vi "event_trager_autoselect.vi"() -> ()   [LabVIEW 2013]
uses:
  <vilib>/silver_ctls/ArrayMatrixCluster/Real Matrix NI_Silver.ctl
  <vilib>/Utility/error.llb/DialogType.ctl
panel:
  in  "Warning Values":dbl[][](array[numeric])
  in  "Check":bool
  in  "repeat 2":dbl=4.0
  in  "interval/min 2":dbl=30.0
  in  "偏置电压":dbl=0.402 format="%0.2p"
  in  "明场周期":dbl=1.0 min=0.0 step=1.0
  in  "扫描起始电压":dbl=-1.0
  in  "振镜步长/um":dbl=0.6
  in  "Volume number":dbl=1.0 min=0.0 step=1.0
  in  "Image number":dbl=200.0
  in  "yx":dbl[][](array[numeric])=[[-0.228, -0.4392], [-0.7848, -0.8083], [-0.6027, 0.1673], [-0.8853, 0.367]]
  in  "waiting_stage/ms":i32=10
  in  "Scan Parameters":T1={"x start"=0.0, "y start"=0.0, "x end"=0.5, "y end"=0.5, "x number"=2.0, "y number"=2.0, "x step"=1.0, "y step"=1.0}
  in  "Stop":bool
  out "illum arr":bool[][](array[boolean])=[[TRUE, FALSE, FALSE, TRUE, FALSE], [FALSE, FALSE, FALSE, FALSE, TRUE], [FALSE, FALSE, FALSE, FALSE, FALSE], [FALSE, FALSE, FALSE, FALSE, TRUE], [FALSE, FALSE, FALSE, TRUE, FALSE]]
  out "total":dbl=4.0
  in  "index":dbl
  in  "exposure/ms":dbl=200.0
  in  "interval/min":dbl=1.0
  in  "repeat":dbl=1.0
  out "y num":dbl=0.772
  out "y target":dbl=-0.228
  out "x num":dbl=0.5608
  out "x target":dbl=-0.4392
  in  "auto compensation":bool
  out "z compensation":T2=[[-1.0, 3.300940438871473, 3.6018808777429463, 1.9028213166144192, 3.2037617554858926, 3.5047021943573657, 4.805642633228839, 7.106583072100312, 6.407523510971785, 5.708463949843258, 6.0094043887147315, 8.310344827586203, 7.611285266457677, 7.912225705329149, 8.213166144200624, 6.514106583072096, 9.81504702194357, 7.115987460815042, 8.416927899686517, 8.717868338557988, 9.018808777429463, 8.319749216300934, 8.620689655172407, 6.9216300940438815, 8.222570532915354, 9.523510971786827, 9.224451410658299, 9.125391849529773, 9.426332288401248, 9.72727272727272], [-0.701298701298701, -0.4017017465293328, -0.10210479175996456, 0.19749216300940375, 0.49708911777877196, 0.7966860725481403, 1.0962830273175084, 1.395879982086877, 1.6954769368562448, 1.9950738916256134, 2.2946708463949816, 2.59426780116435, 2.893864755933718, 3.193461710703086, 3.4930586654724545, 3.7926556202418227, 4.092252575011191, 4.3918495297805595, 4.691446484549928, 4.991043439319295, 5.290640394088664, 5.5902373488580315, 5.8898343036274, 6.189431258396769, 6.4890282131661365, 6.788625167935504, 7.088222122704873, 7.387819077474242, 7.68741603224361, 7.987012987012978], [1.7974025974025984, 2.8956560680698615, 5.193909538737125, 5.492163009404388, 7.790416480071652, 8.088669950738915, 10.38692342140618, 6.685176892073443, 8.983430362740705, 8.28168383340797, 8.579937304075234, 8.878190774742496, 10.176444245409758, 11.474697716077024, 9.972951186744286, 9.971204657411551, 10.569458128078812, 10.667711598746077, 11.96596506941334, 9.264218540080604, 10.562472010747868, 9.86072548141513, 10.158978952082393, 11.457232422749659, 9.955485893416922, 12.053739364084183, 11.35199283475145, 11.650246305418712, 10.948499776085974, 10.246753246753237], [-0.10389610389610282, 0.19301388266905573, 0.48992386923421427, 0.7868338557993728, 1.0837438423645314, 1.38065382892969, 1.6775638154948485, 1.9744738020600072, 2.2713837886251658, 2.5682937751903245, 2.865203761755483, 3.162113748320641, 3.4590237348858, 3.7559337214509583, 4.052843708016117, 4.349753694581276, 4.646663681146434, 4.9435736677115925, 5.240483654276751, 5.537393640841909, 5.834303627407068, 6.131213613972227, 6.4281236005373845, 6.725033587102544, 7.021943573667702, 7.318853560232861, 7.615763546798019, 7.9126735333631775, 8.209583519928337, 8.506493506493495], [4.1948051948051965, 6.49037169726825, 5.785938199731303, 8.081504702194358, 7.377071204657412, 9.672637707120465, 9.968204209583519, 9.263770712046572, 10.559337214509625, 9.855, 11.150470219435732, 10.646036721898785, 12.84160322436184, 12.04, 12.33273622928795, 12.628302731751003, 13.923869234214056, 13.21943573667711, 11.515002239140166, 12.810568741603216, 13.106135244066271, 14.401701746529326, 13.69726824899238, 14.992834751455433, 15.288401253918487, 12.58396775638154, 15.879534258844593, 14.175100761307647, 14.4706672637707, 12.766233766233755], [0.49350649350649545, 0.7877295118674443, 1.0819525302283932, 1.376175548589342, 1.670398566950291, 1.96462158531124, 2.258844603672189, 2.553067622033138, 2.8472906403940863, 3.141513658755036, 3.435736677115985, 3.7299596954769334, 4.024182713837883, 4.318405732198832, 4.6126287505597805, 4.906851768920729, 5.201074787281677, 5.495297805642626, 5.789520824003576, 6.083743842364524, 6.377966860725474, 6.672189879086423, 6.966412897447372, 7.260635915808321, 7.554858934169269, 7.849081952530218, 8.143304970891167, 8.437527989252116, 8.731751007613065, 9.025974025974014], [4.792207792207794, 7.085087326466638, 10.377966860725483, 10.670846394984327, 9.963725929243171, 10.256605463502016, 11.54948499776086, 11.842364532019701, 11.135244066278545, 13.428123600537392, 12.721003134796236, 13.013882669055079, 14.306762203313923, 15.599641737572767, 13.892521271831612, 15.185400806090456, 14.4782803403493, 14.771159874608145, 15.06403940886699, 14.356918943125834, 14.649798477384678, 14.94267801164352, 15.235557545902367, 18.52843708016121, 16.821316614420056, 15.114196148678896, 17.40707568293774, 15.699955217196585, 14.99283475145543, 15.285714285714274], [1.0909090909090935, 1.382445141065833, 1.673981191222572, 1.9655172413793114, 2.2570532915360504, 2.54858934169279, 2.8401253918495293, 3.1316614420062683, 3.4231974921630077, 3.714733542319747, 4.006269592476486, 4.297805642633225, 4.589341692789965, 4.880877742946704, 5.172413793103444, 5.463949843260183, 5.755485893416922, 6.047021943573661, 6.338557993730401, 6.63009404388714, 6.921630094043879, 7.213166144200619, 7.504702194357358, 7.796238244514097, 8.087774294670835, 8.379310344827575, 8.670846394984315, 8.962382445141053, 9.253918495297794, 9.545454545454533], [7.389610389610393, 6.679802955665027, 9.96999552171966, 9.260188087774296, 10.550380653828931, 9.840573219883565, 11.130765785938198, 12.420958351992834, 13.711150918047466, 13.001343484102103, 14.291536050156736, 14.581728616211372, 13.87, 14.2, 14.4, 17.7, 16.0, 15.3, 15.6, 15.9, 15.2, 16.5, 17.8, 17.1, 15.4, 15.6, 15.9, 17.0, 13.5, 14.8], [1.6883116883116918, 1.9771607702642213, 2.266009852216751, 2.5548589341692804, 2.84370801612181, 3.1325570980743396, 3.421406180026869, 3.710255261979399, 3.9991043439319283, 4.287953425884458, 4.576802507836987, 4.8656515897895165, 5.1545006717420465, 5.4433497536945765, 5.732198835647106, 6.0210479175996365, 6.309896999552165, 6.598746081504694, 6.887595163457224, 7.176444245409753, 7.465293327362283, 7.754142409314813, 8.042991491267342, 8.331840573219871, 8.620689655172402, 8.909538737124931, 9.198387819077462, 9.487236901029991, 9.77608598298252, 10.06493506493505], [5.9870129870129905, 7.274518584863416, 6.562024182713841, 7.849529780564264, 7.137035378414691, 8.624540976265116, 9.71204657411554, 9.999552171965965, 11.28705776981639, 12.574563367666816, 16.86206896551724, 14.149574563367665, 13.437080161218088, 13.724585759068514, 14.012091356918937, 14.299596954769363, 15.587102552619788, 16.874608150470213, 16.162113748320635, 15.449619346171062, 15.737124944021486, 14.024630541871911, 17.312136139722334, 17.59964173757276, 15.887147335423187, 15.17465293327361, 17.462158531124036, 18.74966412897446, 15.037169726824885, 13.32467532467531], [2.2857142857142896, 2.5718763994626097, 2.8580385132109294, 3.1442006269592495, 3.430362740707569, 3.7165248544558898, 4.002686968204209, 4.288849081952529, 4.575011195700849, 4.861173309449169, 5.1473354231974895, 5.43349753694581, 5.71965965069413, 6.005821764442449, 6.291983878190769, 6.578145991939088, 6.8643081056874085, 7.150470219435729, 7.436632333184049, 7.722794446932369, 8.008956560680689, 8.295118674429009, 8.58128078817733, 8.86744290192565, 9.15360501567397, 9.43976712942229, 9.725929243170608, 10.012091356918928, 10.298253470667248, 10.584415584415568], [6.584415584415589, 5.8692342140618035, 5.154052843708019, 6.438871473354234, 6.723690103000449, 10.008508732646664, 10.29332736229288, 11.578145991939095, 10.86296462158531, 10.147783251231523, 10.43260188087774, 10.917420510523954, 13.00223914017017, 14.287057769816386, 14.5718763994626, 12.856695029108817, 14.14151365875503, 13.426332288401245, 16.71115091804746, 13.995969547693676, 15.280788177339893, 15.565606806986104, 12.850425436632321, 15.135244066278535, 13.420062695924752, 13.704881325570966, 12.989699955217183, 13.274518584863397, 15.559337214509613, 13.844155844155827], [2.8831168831168883, 3.1665920286609985, 3.4500671742051088, 3.733542319749219, 4.017017465293329, 4.3004926108374395, 4.583967756381551, 4.86744290192566, 5.150918047469769, 5.4343931930138805, 5.717868338557991, 6.001343484102101, 6.284818629646212, 6.568293775190321, 6.851768920734431, 7.135244066278542, 7.418719211822651, 7.702194357366762, 7.985669502910873, 8.269144648454983, 8.552619793999094, 8.836094939543203, 9.119570085087314, 9.403045230631424, 9.686520376175535, 9.969995521719644, 10.253470667263755, 10.536945812807865, 10.820420958351974, 11.103896103896085], [3.181818181818187, 3.4639498432601923, 3.7460815047021976, 4.028213166144203, 4.310344827586208, 4.592476489028215, 4.87460815047022, 5.156739811912225, 5.438871473354231, 5.721003134796236, 6.003134796238242, 6.2852664576802475, 6.567398119122252, 6.849529780564258, 7.131661442006264, 7.41379310344827, 7.695924764890274, 7.978056426332279, 8.260188087774285, 8.54231974921629, 8.824451410658297, 9.106583072100303, 9.388714733542308, 9.670846394984313, 9.952978056426318, 10.235109717868323, 10.51724137931033, 10.799373040752334, 11.08150470219434, 11.363636363636346]]
  in  "Start":bool
  in  "z position":dbl(slide)=-1.0 scale=-75.0..75.0
  out "z":dbl[](array[numeric])=[-1.0, 3.300940438871473, 3.6018808777429463, 1.9028213166144192, 3.2037617554858926, 3.5047021943573657, 4.805642633228839, 7.106583072100312, 6.407523510971785, 5.708463949843258, 6.0094043887147315, 8.310344827586203, 7.611285266457677, 7.912225705329149, 8.213166144200624, 6.514106583072096, 9.81504702194357, 7.115987460815042, 8.416927899686517, 8.717868338557988, 9.018808777429463, 8.319749216300934, 8.620689655172407, 6.9216300940438815, 8.222570532915354, 9.523510971786827, 9.224451410658299, 9.125391849529773, 9.426332288401248, 9.72727272727272, 10.246753246753237, 10.948499776085974, 11.650246305418712, 11.35199283475145, 12.053739364084183, 9.955485893416922, 11.457232422749659, 10.158978952082393, 9.86072548141513, 10.562472010747868, 9.264218540080604, 11.96596506941334, 10.667711598746077, 10.569458128078812, 9.971204657411551, 9.972951186744286, 11.474697716077024, 10.176444245409758, 8.878190774742496, 8.579937304075234, 8.28168383340797, 8.983430362740705, 6.685176892073443, 10.38692342140618, 8.088669950738915, 7.790416480071652, 5.492163009404388, 5.193909538737125, 2.8956560680698615, 1.7974025974025984, 4.1948051948051965, 6.49037169726825, 5.785938199731303, 8.081504702194358, 7.377071204657412, 9.672637707120465, 9.968204209583519, 9.263770712046572, 10.559337214509625, 9.855, 11.150470219435732, 10.646036721898785, 12.84160322436184, 12.04, 12.33273622928795, 12.628302731751003, 13.923869234214056, 13.21943573667711, 11.515002239140166, 12.810568741603216, 13.106135244066271, 14.401701746529326, 13.69726824899238, 14.992834751455433, 15.288401253918487, 12.58396775638154, 15.879534258844593, 14.175100761307647, 14.4706672637707, 12.766233766233755, 15.285714285714274, 14.99283475145543, 15.699955217196585, 17.40707568293774, 15.114196148678896, 16.821316614420056, 18.52843708016121, 15.235557545902367, 14.94267801164352, 14.649798477384678, 14.356918943125834, 15.06403940886699, 14.771159874608145, 14.4782803403493, 15.185400806090456, 13.892521271831612, 15.599641737572767, 14.306762203313923, 13.013882669055079, 12.721003134796236, 13.428123600537392, 11.135244066278545, 11.842364532019701, 11.54948499776086, 10.256605463502016, 9.963725929243171, 10.670846394984327, 10.377966860725483, 7.085087326466638, 4.792207792207794, 7.389610389610393, 6.679802955665027, 9.96999552171966, 9.260188087774296, 10.550380653828931, 9.840573219883565, 11.130765785938198, 12.420958351992834, 13.711150918047466, 13.001343484102103, 14.291536050156736, 14.581728616211372, 13.87, 14.2, 14.4, 17.7, 16.0, 15.3, 15.6, 15.9, 15.2, 16.5, 17.8, 17.1, 15.4, 15.6, 15.9, 17.0, 13.5, 14.8, 13.32467532467531, 15.037169726824885, 18.74966412897446, 17.462158531124036, 15.17465293327361, 15.887147335423187, 17.59964173757276, 17.312136139722334, 14.024630541871911, 15.737124944021486, 15.449619346171062, 16.162113748320635, 16.874608150470213, 15.587102552619788, 14.299596954769363, 14.012091356918937, 13.724585759068514, 13.437080161218088, 14.149574563367665, 16.86206896551724, 12.574563367666816, 11.28705776981639, 9.999552171965965, 9.71204657411554, 8.624540976265116, 7.137035378414691, 7.849529780564264, 6.562024182713841, 7.274518584863416, 5.9870129870129905, 6.584415584415589, 5.8692342140618035, 5.154052843708019, 6.438871473354234, 6.723690103000449, 10.008508732646664, 10.29332736229288, 11.578145991939095, 10.86296462158531, 10.147783251231523, 10.43260188087774, 10.917420510523954, 13.00223914017017, 14.287057769816386, 14.5718763994626, 12.856695029108817, 14.14151365875503, 13.426332288401245, 16.71115091804746, 13.995969547693676, 15.280788177339893, 15.565606806986104, 12.850425436632321, 15.135244066278535, 13.420062695924752, 13.704881325570966, 12.989699955217183, 13.274518584863397, 15.559337214509613, 13.844155844155827]
  out "xy":dbl[][](array[numeric])=[[0.0, 0.0], [0.0, 1.0], [1.0, 1.0], [1.0, 0.0]]
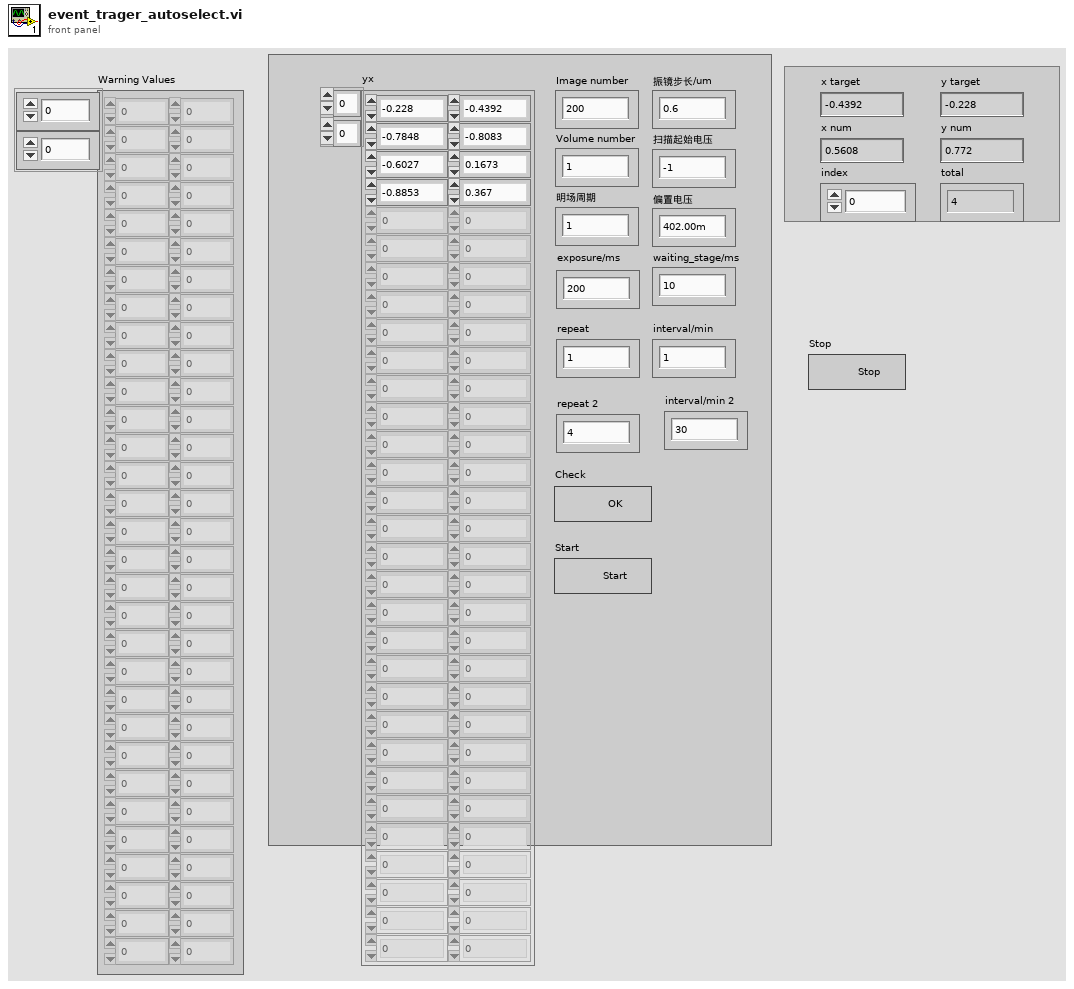
[diagram p1: front panel]
types:
  T1 = cluster{"x start":dbl, "y start":dbl, "x end":dbl, "y end":dbl, "x number":dbl, "y number":dbl, "x step":dbl, "y step":dbl}
  T2 = typedef "Real Matrix NI_Silver.ctl" = dbl[][]
  T3 = typedef "DialogType.ctl" = u16
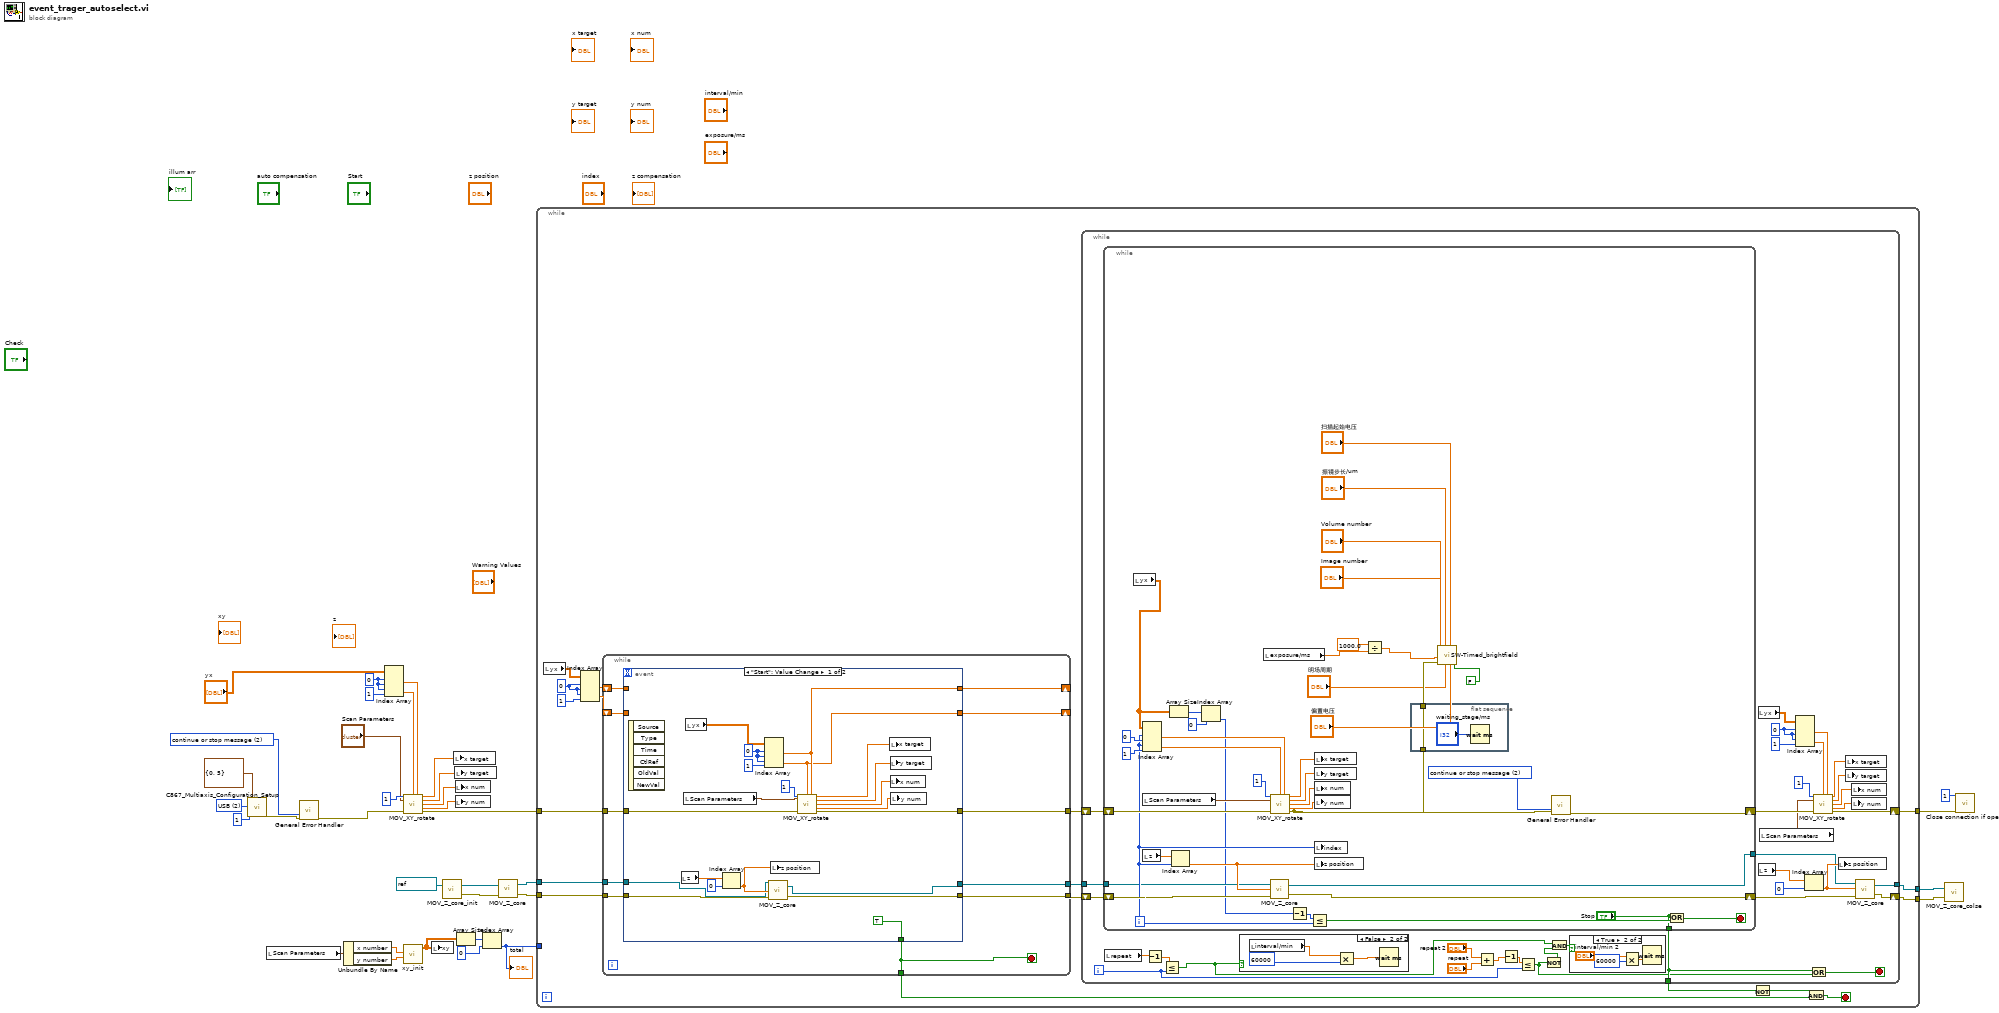
[diagram p0: block diagram]
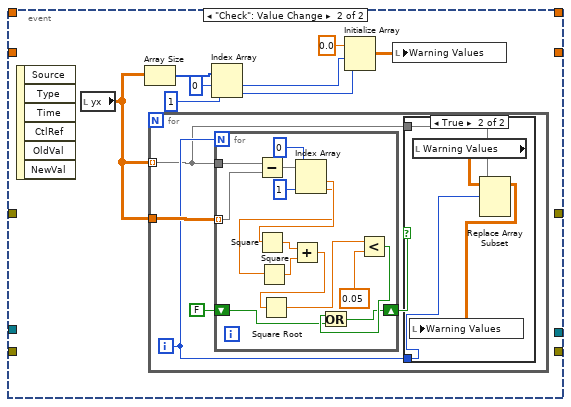
[diagram p4: hidden frame]
diagram:
  w3 = T3 2 items=["no dialog", "OK message", "continue or stop message", "OK message + warnings", "continue/stop + warnings"] ("type of dialog (OK msg:1)")
  w8 = u16 2 items=["RS232", "RS232 DaisyChain", "USB"] ("Interface")
  w13 = 0
  n1 = call "C867_Multiaxis_Configuration_Setup.vi"("System no."=1, "Interface"=w8, "RS232 settings"=cluster{"Portnumber":i32, "Baudrate":u16} {"Portnumber"=0, "Baudrate"=5}) -> ("error out"=w5:errorcluster)  [unwired: 10 in, 6 out]
  n2 = local read "Scan Parameters"() -> (w18:T1)
  n3 = call <vilib>:"General Error Handler.vi"("type of dialog (OK msg:1)"=w3, "error in (no error)"=w5) -> ("error out"=w4:errorcluster)  [unwired: 9 in, 4 out]
  n4 = Unbundle By Name(w18) -> ("x number"=w17:dbl, "y number"=w16:dbl)
  n5 = Index Array(array="yx", index (row) #1=w13, index (col) #1=w13, index (row) #2=w13, index (col) #2=1) -> (element #1=w10:dbl, element #2=w9:dbl)
  n6 = call "MOV_XY_rotate.vi"("System no."=1, "x state"=w9, "y state"=w10, "param"="Scan Parameters", "error in"=w4) -> ("x target"=w28:dbl, "y target"=w29:dbl, "x num out"=w30:dbl, "y num out"=w31:dbl, "error out"=w32:errorcluster)  [unwired: 6 in]
  n7 = call "xy_init.vi"("y number"=w16, "x number"=w17) -> ("xy"=w25:dbl[][])  [unwired: 9 in]
  n8 = local write "xy"(w25) -> ()
  n9 = call "MOV_Z_core_init.vi"("VISA resource name"=refnum<visa-resource-name> "COM8") -> ("error out"=w34:errorcluster, "VISA resource name out"=w23:refnum<visa-resource-name>)  [unwired: 1 in]
  n10 = local write "x target"(w28) -> ()
  n11 = local write "y target"(w29) -> ()
  n12 = local write "x num"(w30) -> ()
  n13 = local write "y num"(w31) -> ()
  n14 = Array Size(array=w25) -> (size(s)=w27:i32[])
  n15 = Index Array(array=w27, index=0) -> (element=w14:i32)
  "total" <- w14
  n16 = call "MOV_Z_core.vi"("error in (no error)"=w34, "VISA resource name"=w23) -> ("error out"=w33:errorcluster, "VISA resource name out"=w22:refnum<visa-resource-name>)  [unwired: 1 in]
  n17 = while {
    tunnel: w33 -> [w51]
    tunnel: w32 -> [w50]
    tunnel: w22 -> [w39]
    tunnel: [w37] -> w21
    tunnel: [w36] -> w20
    tunnel: w14 -> [_]
    tunnel: [w35] -> w1
    stop <- w40 stop-if-true
    w46 = 0
    n18 = local read "yx"() -> (w47:dbl[][])
    n19 = Index Array(array=w47, index (row) #1=w46, index (col) #1=w46, index (row) #2=w46, index (col) #2=1) -> (element #1=w45:dbl, element #2=w44:dbl)
    n20 = while {
      shift-right: [w137] -> _
      shift-left: w44 -> [w146]
      shift-right: [w141] -> _
      shift-left: w45 -> [w147]
      tunnel: w50 -> [w142]
      tunnel: [w143] -> w52
      tunnel: w51 -> [w145]
      tunnel: [w144] -> w49
      tunnel: [w138] -> w43
      tunnel: w39 -> [w140]
      tunnel: [w139] -> w38
      stop <- w138 stop-if-true
      n21 = event shown="[0] \"Start\": Value Change" {
        selector: _ -> [_ _]
        dyn-events: _ -> [_ _]
        timeout: _ -> [_ _]
        tunnel: w147 -> [_ _]
        tunnel: [w153 _] -> w141
        tunnel: w146 -> [_ _]
        tunnel: [w152 _] -> w137
        tunnel: [TRUE _] -> w138
        tunnel: w145 -> [w165 _]
        tunnel: [w164 _] -> w144
        tunnel: [w166 _] -> w143
        tunnel: w142 -> [w167 _]
        tunnel: w140 -> [w151 _]
        tunnel: [w150 _] -> w139
        event "Start": Value Change {
          w158 = 0
          n22 = event-data() -> ()  [unwired: 1 in, 6 out]
          n23 = local read "z"() -> (w154:dbl[])
          n24 = local read "Scan Parameters"() -> (w148:T1)
          n25 = local read "yx"() -> (w159:dbl[][])
          n26 = Index Array(array=w154, index=0) -> (element=w155:dbl)
          n27 = Index Array(array=w159, index (row) #1=w158, index (col) #1=w158, index (row) #2=w158, index (col) #2=1) -> (element #1=w153:dbl, element #2=w152:dbl)
          n28 = call "MOV_Z_core.vi"("error in (no error)"=w165, "数据值"=w155, "VISA resource name"=w151) -> ("error out"=w164:errorcluster, "VISA resource name out"=w150:refnum<visa-resource-name>)
          n29 = local write "z position"(w155) -> ()
          n30 = call "MOV_XY_rotate.vi"("System no."=1, "x state"=w152, "y state"=w153, "param"=w148, "error in"=w167) -> ("x target"=w163:dbl, "y target"=w162:dbl, "x num out"=w161:dbl, "y num out"=w160:dbl, "error out"=w166:errorcluster)  [unwired: 6 in]
          n31 = local write "x target"(w163) -> ()
          n32 = local write "y target"(w162) -> ()
          n33 = local write "x num"(w161) -> ()
          n34 = local write "y num"(w160) -> ()
        }
        event "Check": Value Change {
          n35 = event-data() -> ()  [unwired: 1 in, 6 out]
          n36 = local read "yx"() -> (w176:dbl[][])
          n37 = Array Size(array=w176) -> (size(s)=w174:i32[])
          n38 = for {
            tunnel: w176 -> [w178] mode=indexing
            tunnel: w176 -> [w181]
            i -> [w179]
            n39 = for {
              N: w179 -> [_]
              tunnel: w181 -> [w199] mode=indexing
              tunnel: w178 -> [w200]
              shift-right: [w186] -> w177
              shift-left: FALSE -> [w187]
              n40 = Subtract(x=w200, y=w199) -> (x-y=w198:dbl[])
              n41 = Index Array(array=w198, index #1=0 ("index"), index #2=1 ("index")) -> (element #1=w195:dbl, element #2=w194:dbl)
              n42 = Square(x=w195) -> (x^2=w193:dbl)
              n43 = Square(x=w194) -> (x^2=w192:dbl)
              n44 = Add(x=w193, y=w192) -> (x+y=w191:dbl)
              n45 = Square Root(x=w191) -> (sqrt(x)=w190:dbl)
              n46 = Less?(x=w190, y=0.05) -> (x < y?=w188:bool)
              n47 = Or(x=w188, y=w187) -> (x .or. y?=w186:bool)
            }
            n48 = case shown="True" w177 {
              tunnel: w179 -> [_ w184]
              tunnel: w178 -> [_ w183]
              frame False {
              }
              frame True {
                n49 = local read "Warning Values"() -> (w185:dbl[][])
                n50 = Replace Array Subset(array=w185, new element=w183, index (row)=w184) -> (w182:dbl[][])  [unwired: 1 in]
                n51 = local write "Warning Values"(w182) -> ()
              }
            }
          }
          n52 = Index Array(array=w174, index #1=0 ("index"), index #2=1 ("index")) -> (element #1=w171:i32, element #2=w170:i32)
          n53 = Initialize Array(0.0 ("element"), w171, w170) -> (w169:dbl[][])
          n54 = local write "Warning Values"(w169) -> ()
        }
      }
    }
    n55 = while {
      shift-right: [w86] -> w35
      shift-left: w52 -> [w88]
      shift-right: [w85] -> w36
      shift-left: w49 -> [w87]
      tunnel: [w69] -> w42
      tunnel: w38 -> [w66]
      tunnel: [w64] -> w37
      i -> [w57]
      stop <- w70 stop-if-true
      w71 = 0
      n56 = while {
        shift-right: [w93] -> w76
        shift-left: w88 -> [w131]
        shift-right: [w112] -> w78
        shift-left: w87 -> [w130]
        tunnel: ["Stop"] -> w69
        tunnel: w66 -> [w115]
        tunnel: [w113] -> w65
        i -> [w118]
        stop <- w119 stop-if-true
        w92 = T3 2 items=["no dialog", "OK message", "continue or stop message", "OK message + warnings", "continue/stop + warnings"] ("type of dialog (OK msg:1)")
        n57 = local read "yx"() -> (w106:dbl[][])
        n58 = local read "Scan Parameters"() -> (w110:T1)
        n59 = Index Array(array=w106, index (row) #1=w118, index (col) #1=0, index (row) #2=w118, index (col) #2=1) -> (element #1=w128:dbl, element #2=w127:dbl)
        n60 = local read "z"() -> (w126:dbl[])
        n61 = Array Size(array=w106) -> (size(s)=w109:i32[])
        n62 = Index Array(array=w126, index=w118) -> (element=w121:dbl)
        n63 = Index Array(array=w109, index=0) -> (element=w107:i32)
        n64 = local read "exposure/ms"() -> (w98:dbl)
        n65 = call "MOV_Z_core.vi"("error in (no error)"=w130, "数据值"=w121, "VISA resource name"=w115) -> ("error out"=w112:errorcluster, "VISA resource name out"=w113:refnum<visa-resource-name>)
        n66 = call "MOV_XY_rotate.vi"("System no."=1, "x state"=w127, "y state"=w128, "param"=w110, "error in"=w131) -> ("x target"=w125:dbl, "y target"=w124:dbl, "x num out"=w123:dbl, "y num out"=w122:dbl, "error out"=w94:errorcluster)  [unwired: 6 in]
        n67 = Decrement(x=w107) -> (x-1=w116:i32)
        n68 = Less Or Equal?(x=w116, y=w118) -> (x <= y?=w117:bool)
        n69 = local write "x target"(w125) -> ()
        n70 = local write "y target"(w124) -> ()
        n71 = local write "x num"(w123) -> ()
        n72 = local write "y num"(w122) -> ()
        n73 = local write "index"(w118) -> ()
        n74 = local write "z position"(w121) -> ()
        n75 = Divide(x=1000.0, y=w98) -> (x/y=w96:dbl)
        n76 = flat-sequence {
          tunnel: w94 -> [w132]
          tunnel: [w132] -> w105
          frame #0 {
            n77 = Wait (ms)(milliseconds to wait="waiting_stage/ms") -> ()  [unwired: 1 out]
          }
        }
        n78 = call "SW-Timed_brightfield.vi"("Flip Z"=FALSE, "偏置电压"="偏置电压", "扫描起始电压"="扫描起始电压", "明场周期"="明场周期", "振镜步长/um"="振镜步长/um", "error in (no error)"=w105, "荧光帧率/Hz"=w96, "Image number"="Image number", "Volume number"="Volume number") -> ()  [unwired: 3 in]
        n79 = call <vilib>:"General Error Handler.vi"("type of dialog (OK msg:1)"=w92, "error in (no error)"=w94) -> ("error out"=w93:errorcluster)  [unwired: 9 in, 4 out]
        n80 = Or(x="Stop", y=w117) -> (x .or. y?=w119:bool)
      }
      n81 = local read "repeat"() -> (w67:dbl)
      n82 = Decrement(x=w67) -> (x-1=w68:dbl)
      n83 = Less Or Equal?(x=w68, y=w57) -> (x <= y?=w54:bool)
      n84 = case shown="False" w54 {
        frame True {
        }
        frame False {
          n85 = local read "interval/min"() -> (w136:dbl)
          n86 = Multiply(x=w136, y=60000) -> (x*y=w134:dbl)
          n87 = Wait (ms)(milliseconds to wait=w134) -> ()  [unwired: 1 out]
        }
      }
      n88 = Add(x="repeat 2", y="repeat") -> (x+y=w59:dbl)
      n89 = Decrement(x=w59) -> (x-1=w58:dbl)
      n90 = Less Or Equal?(x=w58, y=w57) -> (x <= y?=w56:bool)
      n91 = Not(x=w56) -> (.not. x?=w55:bool)
      n92 = And(x=w54, y=w55) -> (x .and. y?=w53:bool)
      n93 = case shown="True" w53 {
        frame False {
        }
        frame True {
          n94 = Multiply(x="interval/min 2", y=60000) -> (x*y=w89:dbl)
          n95 = Wait (ms)(milliseconds to wait=w89) -> ()  [unwired: 1 out]
        }
      }
      n96 = local read "yx"() -> (w74:dbl[][])
      n97 = local read "z"() -> (w84:dbl[])
      n98 = local read "Scan Parameters"() -> (w62:T1)
      n99 = Index Array(array=w74, index (row) #1=w71, index (col) #1=w71, index (row) #2=w71, index (col) #2=1) -> (element #1=w72:dbl, element #2=w73:dbl)
      n100 = Index Array(array=w84, index=0) -> (element=w77:dbl)
      n101 = Or(x=w69, y=w56) -> (x .or. y?=w70:bool)
      n102 = call "MOV_XY_rotate.vi"("System no."=1, "x state"=w73, "y state"=w72, "param"=w62, "error in"=w76) -> ("x target"=w79:dbl, "y target"=w80:dbl, "x num out"=w81:dbl, "y num out"=w82:dbl, "error out"=w86:errorcluster)  [unwired: 6 in]
      n103 = local write "z position"(w77) -> ()
      n104 = local write "x target"(w79) -> ()
      n105 = local write "y target"(w80) -> ()
      n106 = local write "x num"(w81) -> ()
      n107 = local write "y num"(w82) -> ()
      n108 = call "MOV_Z_core.vi"("error in (no error)"=w78, "数据值"=w77, "VISA resource name"=w65) -> ("error out"=w85:errorcluster, "VISA resource name out"=w64:refnum<visa-resource-name>)
    }
    n109 = Not(x=w42) -> (.not. x?=w41:bool)
    n110 = And(x=w41, y=w43) -> (x .and. y?=w40:bool)
  }
  n111 = call "MOV_Z_core_colse.vi"("error in (no error)"=w20, "VISA resource name"=w21) -> ()  [unwired: 1 in]
  n112 = call "Close connection if open.vi"("System no."=1, "error in"=w1) -> ()  [unwired: 1 in, 17 out]
